vi "Create New Path File.vi"() -> ()   [LabVIEW 2020]
uses:
  Framework/Robot Global Data.vi
panel:
  out "deleted path":path
  out "error out":errorcluster
  out "path":path
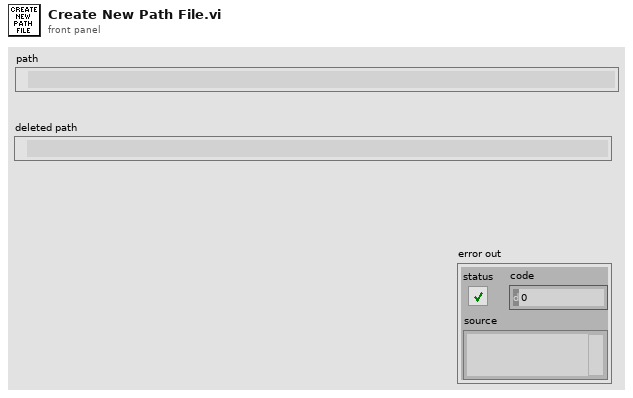
[diagram p1: front panel]
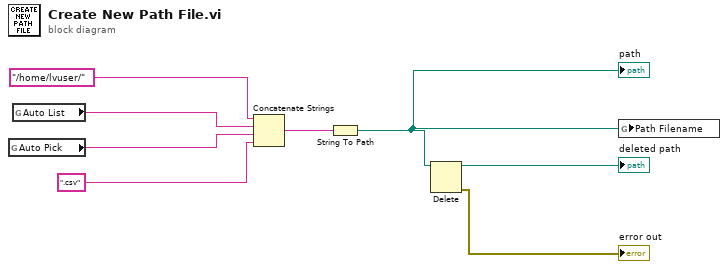
[diagram p0: block diagram]
diagram:
  n1 = global read "Robot Global Data.vi" "Auto Pick"() -> (w4:string)
  n2 = global read "Robot Global Data.vi" "Auto List"() -> (w5:string)
  n3 = Concatenate Strings("/home/lvuser/", w5, w4, ".csv") -> (w6:string)
  n4 = String To Path(string=w6) -> (path=w3:path)
  "path" <- w3
  n5 = Delete(path (use dialog)=w3) -> (deleted path=→"deleted path":path, error out=→"error out":errorcluster)  [unwired: 4 in, 1 out]
  n6 = global write "Robot Global Data.vi" "Path Filename"(w3) -> ()
